vi "Get Data.vi"(8 "error in":errorcluster, 11 "Yokogawa in":refnum<class "Yokogawa.lvclass">) -> (0 "error out":errorcluster, 2 "Data Out":T1[](array[typedef]), 3 "Yokogawa out":refnum<class "Yokogawa.lvclass">)   [LabVIEW 2015, in "Yokogawa.lvclass"]
uses:
  Yokogawa.lvclass
  Parent/Power Data.ctl
  Parent/Power Meter.lvclass/Power Meter.ctl
  Parent/Read Address.vi
  Parent/Power Meter.lvclass
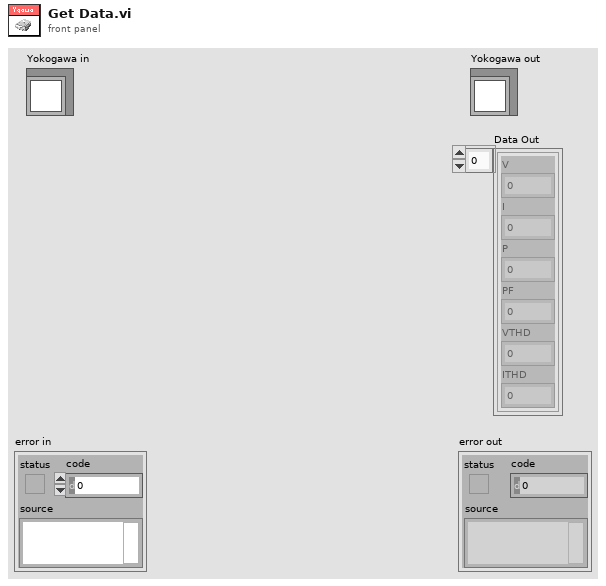
[diagram p1: front panel]
types:
  T1 = typedef "Power Meter.lvclass/Power Data.ctl" = cluster{"V":dbl, "I":dbl, "P":dbl, "PF":dbl, "VTHD":dbl, "ITHD":dbl}
  T2 = cluster{"[0]":dbl, "[1]":dbl, "[2]":dbl, "[3]":dbl, "[4]":dbl, "[5]":dbl}
  T3 = cluster{"[0]":dbl, "[1]":dbl, "[2]":dbl, "[3]":dbl, "[4]":dbl, "[5]":dbl}[]
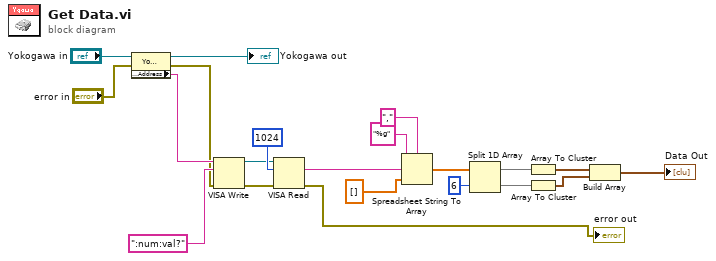
[diagram p0: block diagram]
diagram:
  n1 = property class="Yokogawa.lvclass"(reference="Yokogawa in", error in="error in") -> (reference out=→"Yokogawa out":refnum<class "Yokogawa.lvclass">, error out=w2:errorcluster, "Accessors:Address"=w4:string)
  n2 = VISA Write(VISA resource name=w4, write buffer=":num:val?", error in (no error)=w2) -> (VISA resource name out=w16:refnum<visa-resource-name>, error out=w15:errorcluster)  [unwired: 1 out]
  n3 = VISA Read(VISA resource name=w16, byte count=u32 1024, error in (no error)=w15) -> (read buffer=w13:string, error out=→"error out":errorcluster)  [unwired: 2 out]
  n4 = Spreadsheet String To Array(delimiter (Tab)=",", format string="%g" ("delimiter (Tab)"), spreadsheet string=w13, array type (2D Dbl)=dbl[] []) -> (array=w10:dbl[])
  n5 = Split 1D Array(array=w10, index=6) -> (first subarray=w20:dbl[], second subarray=w19:dbl[])
  n6 = Array To Cluster(array=w20) -> (cluster=w9:T2)
  n7 = Array To Cluster(array=w19) -> (cluster=w8:T2)
  n8 = Build Array(w9, w8) -> (→"Data Out":T3)
